vi "TunePID.vi"(8 "error in (no error)":errorcluster) -> ()   [LabVIEW 2014]
panel:
  out "error out":errorcluster
  in  "Position PID":cluster{"P":dbl, "I":dbl, "D":dbl}={"P"=1.0, "I"=0.0, "D"=0.0}
  out "Position":T1(graph)
  in  "Speed PID":cluster{"P":dbl, "I":dbl, "D":dbl}={"P"=1.0, "I"=0.0, "D"=0.0}
  out "Speed":T1(graph)
  in  "Set Speed PID":bool
  in  "Set Position PID":bool
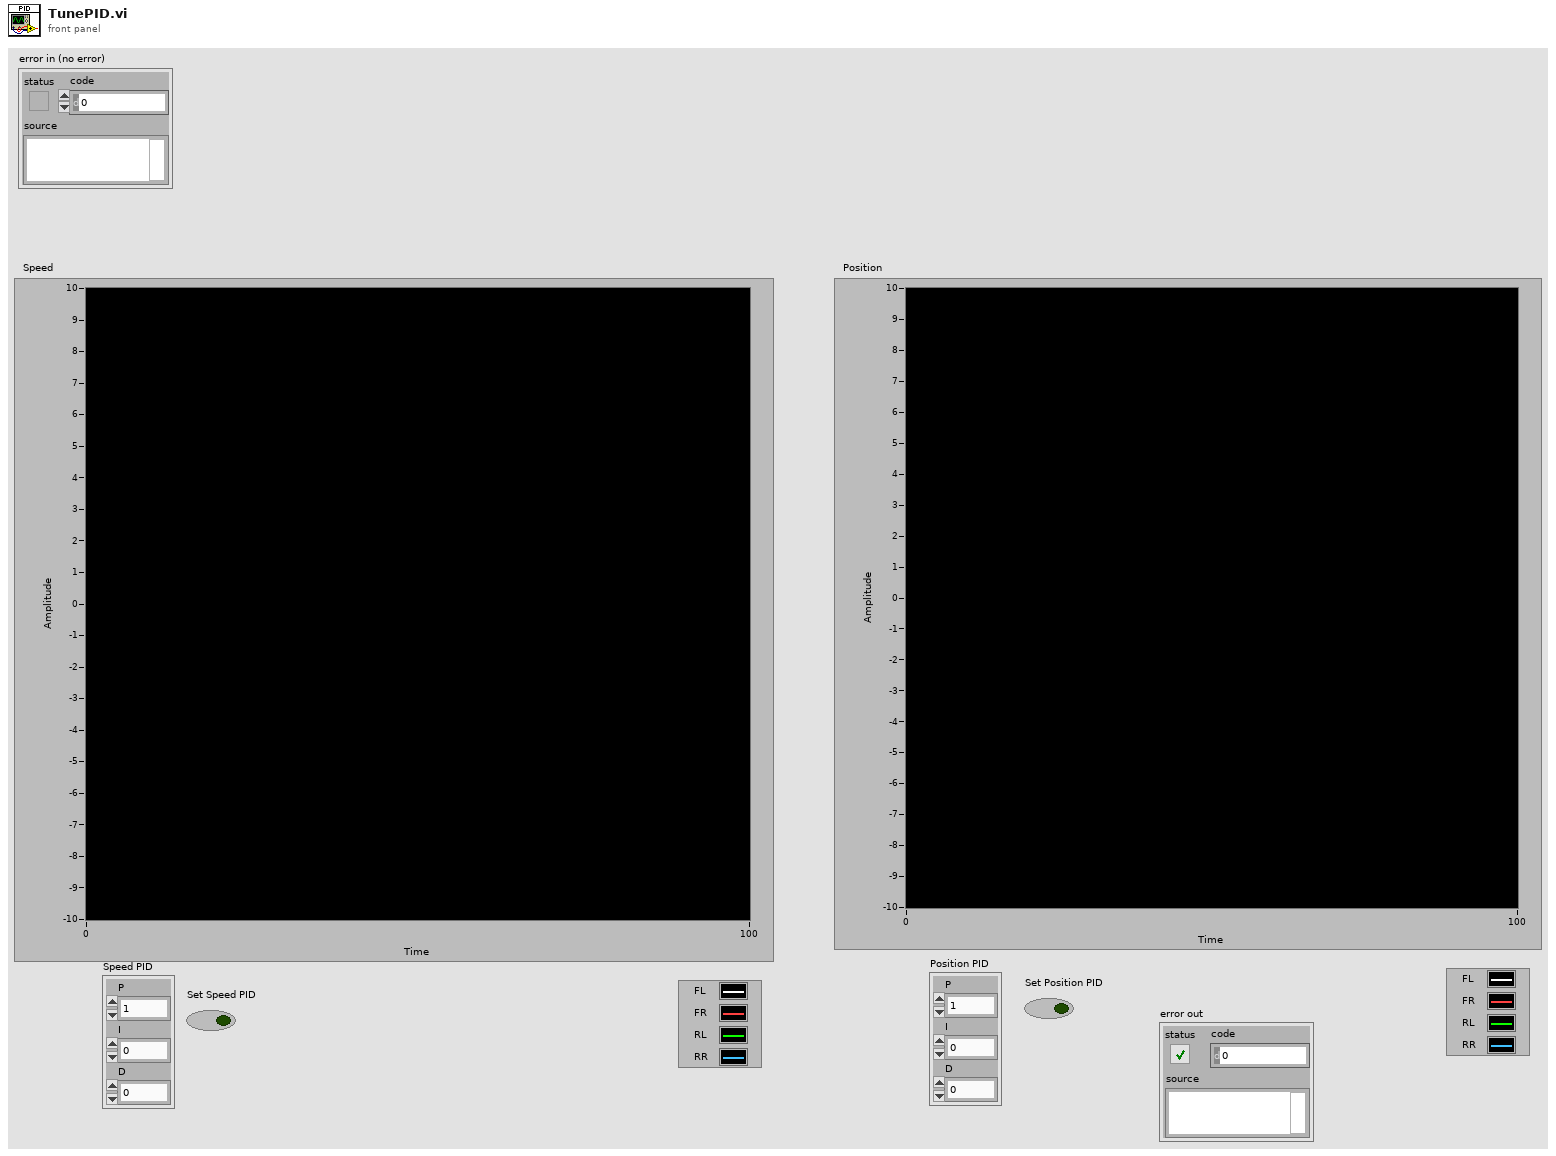
[diagram p1: front panel]
types:
  T1 = cluster{"[0]":dbl, "[1]":dbl, "[2]":dbl, "[3]":dbl, "[4]":dbl, "[5]":dbl, "[6]":dbl, "[7]":dbl, "[8]":dbl}
  T2 = typedef "WPI_MotorControlDeviceRef.ctl" = cluster{"DeviceStatus":errorcluster, "Type":T3, "PWM":cluster{"Controller":T4, "PWM Channel":T5, "DeadBand":T6}, "CAN":cluster{"Device Number":u8, "Control Mode":T7, "Semaphore":T8, "Max Vout":dbl, "TalonSRX Control Mode":T9}, "Invert":bool, "TransformRef":T10, "InvTransformRef":T10}
  T3 = typedef "WPI_MotorControlType.ctl" = enum16{"PWM", "CAN", "CANTalonSRX"}
  T4 = typedef "FPGA_TypedefDigitalModule.ctl" = enum16{"Controller 1"}
  T5 = typedef "FPGA_DIOPWMChannel.ctl" = enum8{"PWM 0", "PWM 1", "PWM 2", "PWM 3", "PWM 4", "PWM 5", "PWM 6", "PWM 7", "PWM 8", "PWM 9", "PWM MXP 0", "PWM MXP 1", "PWM MXP 2", "PWM MXP 3", "PWM MXP 4", "PWM MXP 5", "PWM MXP 6", "PWM MXP 7", "PWM MXP 8", "PWM MXP 9", "Invalid"}
  T6 = typedef "WPI_PWMDeadband.ctl" = cluster{"Name":string, "maxPositivePwm":i32, "minPositivePwm":i32, "centerPwm":i32, "maxNegativePwm":i32, "minNegativePwm":i32, "angularRange":u16}
  T7 = typedef "WPI_CANJaguar_ControlMode.ctl" = enum8{"Percent VBus", "Current", "Speed", "Position", "Voltage"}
  T8 = typedef "Semaphore RefNum" = refnum<k1>
  T9 = typedef "WPI_CANTalonSRX_APIControlMode.ctl" = enum8{"Percent VBus", "Speed", "Position", "Slave", "Unchanged / Invalid"}
  T10 = typedef "WPI_PWMTransform_ConPane.ctl" = refnum<vi>
  T11 = typedef "WPI_CANTalonSRX_GlobalStatus.ctl" = cluster{"Applied Throttle":dbl, "Module Enabled":bool, "CAN Error":errorcluster, "Closed Loop Error":dbl, "Forward Limit Switch Closed":bool, "Reverse Limit Switch Closed":bool, "Sensor Position":dbl, "Sensor Velocity":dbl, "Current":dbl, "Sticky Fault - Over Temp":bool, "Sticky Fault - Under Voltage":bool, "Sticky Fault - Forward Limit":bool, "Sticky Fault - Reverse Limit":bool, "Sticky Fault - Forward Soft Limit":bool, "Sticky Fault - Reverse Soft Limit":bool, "Brake is Enabled":bool, "Encoder Position":dbl, "Encoder Velocity":dbl, "Encoder Index Count":dbl, "Encoder A Pin State":bool, "Encoder B Pin State":bool, "Encoder Index Pin State":bool, "Analog In":dbl, "Analog In Velocity":dbl, "Temperature (C)":dbl, "Battery Voltage":dbl}
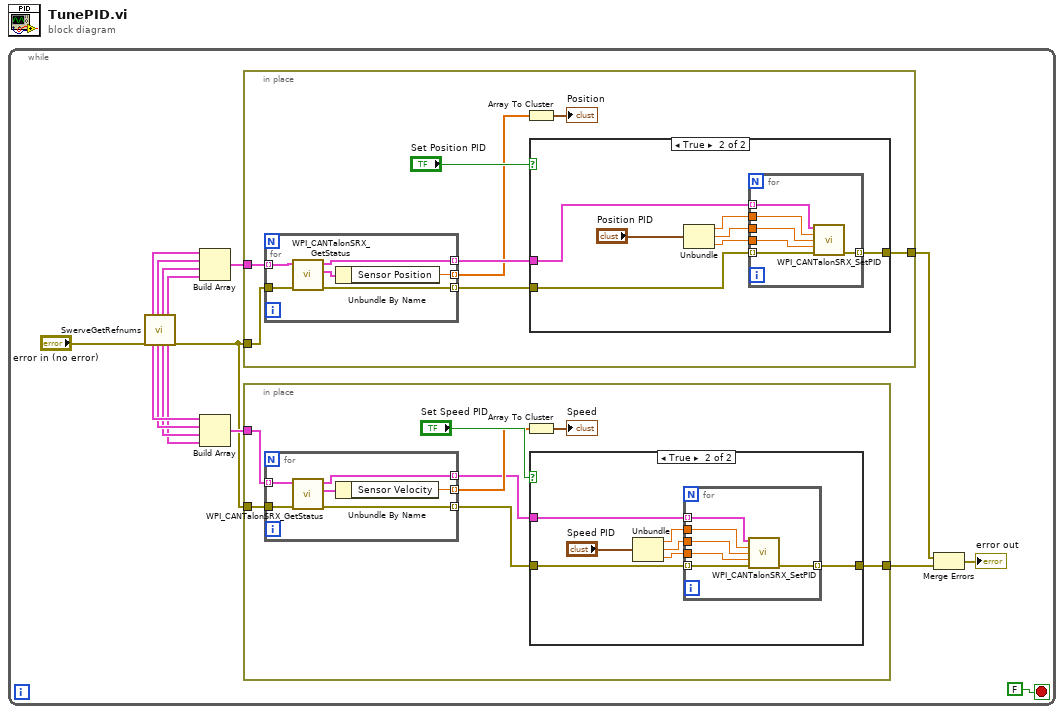
[diagram p0: block diagram]
diagram:
  n1 = while {
    stop <- FALSE stop-if-true
    n2 = call "SwerveGetRefnums.vi"("error in (no error)"="error in (no error)") -> ("FL Steering"=w9:T2, "FL Speed"=w14:T2, "FR Steering"=w8:T2, "FR Speed"=w13:T2, "RL Steering"=w7:T2, "RL Speed"=w12:T2, "RR Steering"=w6:T2, "RR Speed"=w11:T2, "error out"=w4:errorcluster)  [unwired: 10 in]
    n3 = Build Array(w9, w8, w7, w6) -> (w5:T2[])
    n4 = Build Array(w14, w13, w12, w11) -> (w10:T2[])
    n5 = in-place {
      in-place-border: w5 -> [w21]
      in-place-border: w4 -> [w23]
      in-place-border: [w19] -> w3
      n6 = for {
        tunnel: w21 -> [w30] mode=indexing
        tunnel: [w28] -> w18 mode=indexing
        tunnel: w23 -> [w27]
        tunnel: [w26] -> w22 mode=indexing
        tunnel: [w25] -> w20 mode=indexing
        n7 = call <vilib>:"WPI_CANTalonSRX_GetStatus.vi"("error in (no error)"=w27, "CAN Talon SRX Ref"=w30) -> ("error out"=w26:errorcluster, "Talon SRX Status"=w29:T11, "CAN Talon SRX Ref Out"=w25:T2)  [unwired: 7 in]
        n8 = Unbundle By Name(w29) -> ("Sensor Position"=w28:dbl)
      }
      n9 = Array To Cluster(array=w18) -> (cluster=→"Position":T1)
      n10 = case shown="True" "Set Position PID" {
        tunnel: w20 -> [_ w38]
        tunnel: w22 -> [w31 w33]
        tunnel: [w31 w32] -> w19
        frame False {
        }
        frame True {
          n11 = Unbundle("Position PID") -> ("P"=w37:dbl, "I"=w36:dbl, "D"=w34:dbl)
          n12 = for {
            tunnel: w38 -> [w44] mode=indexing
            tunnel: w37 -> [w43]
            tunnel: w36 -> [w42]
            tunnel: w34 -> [w41]
            tunnel: w33 -> [w40] mode=indexing
            tunnel: [w39] -> w32 mode=indexing
            n13 = call <vilib>:"WPI_CANTalonSRX_SetPID.vi"("CAN Talon SRX Ref"=w44, "P"=w43, "I"=w42, "D"=w41, "error in (no error)"=w40) -> ("error out"=w39:errorcluster)  [unwired: 9 in, 1 out]
          }
        }
      }
    }
    n14 = in-place {
      in-place-border: w10 -> [w48]
      in-place-border: w4 -> [w50]
      in-place-border: [w46] -> w2
      n15 = for {
        tunnel: w48 -> [w58] mode=indexing
        tunnel: [w56] -> w51 mode=indexing
        tunnel: w50 -> [w55]
        tunnel: [w54] -> w49 mode=indexing
        tunnel: [w53] -> w47 mode=indexing
        n16 = call <vilib>:"WPI_CANTalonSRX_GetStatus.vi"("error in (no error)"=w55, "CAN Talon SRX Ref"=w58) -> ("error out"=w54:errorcluster, "Talon SRX Status"=w57:T11, "CAN Talon SRX Ref Out"=w53:T2)  [unwired: 7 in]
        n17 = Unbundle By Name(w57) -> ("Sensor Velocity"=w56:dbl)
      }
      n18 = Array To Cluster(array=w51) -> (cluster=→"Speed":T1)
      n19 = case shown="True" "Set Speed PID" {
        tunnel: w47 -> [_ w66]
        tunnel: w49 -> [w59 w61]
        tunnel: [w59 w60] -> w46
        frame False {
        }
        frame True {
          n20 = Unbundle("Speed PID") -> ("P"=w65:dbl, "I"=w64:dbl, "D"=w62:dbl)
          n21 = for {
            tunnel: w66 -> [w72] mode=indexing
            tunnel: w65 -> [w71]
            tunnel: w64 -> [w70]
            tunnel: w62 -> [w69]
            tunnel: w61 -> [w68] mode=indexing
            tunnel: [w67] -> w60 mode=indexing
            n22 = call <vilib>:"WPI_CANTalonSRX_SetPID.vi"("CAN Talon SRX Ref"=w72, "P"=w71, "I"=w70, "D"=w69, "error in (no error)"=w68) -> ("error out"=w67:errorcluster)  [unwired: 9 in, 1 out]
          }
        }
      }
    }
    n23 = Merge Errors(w3, w2) -> (→"error out":errorcluster)
  }
